vi "Set Browse Start Path.vi"(10 "Start Path":path=path "D:/gitlab/imponator-series-actor/CFGs", 11 "File Provider in":refnum<class "File Provider.lvclass">) -> (3 "File Provider out":refnum<class "File Provider.lvclass">)   [LabVIEW 2024, in "File Provider.lvlib" / "File Provider.lvclass"]
uses:
  File Provider.lvclass
  File Provider.lvclass/File Provider.ctl
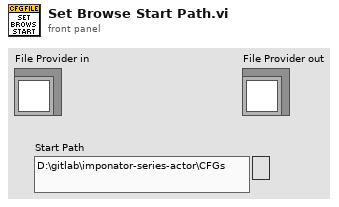
[diagram p1: front panel]
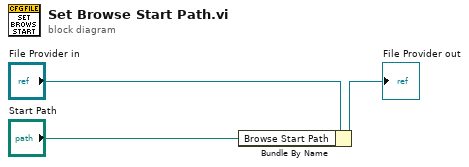
[diagram p0: block diagram]
diagram:
  n1 = Bundle By Name(cluster="File Provider in", "Browse Start Path"="Start Path") -> (→"File Provider out":refnum<class "File Provider.lvclass">)
